vi "THzTimeScan_830_PSD_TA_170222.vi"(0 "input":T1={"Step Number"=0, "Step"=0.0, "Start Position"=0.0, "Time-out"=0, "Lockin Address"="", "Short term \nAverage#"=0, 0, "ESP300 Axis"=0, "Value"="", "Delay"=0.0, "Delay2"=0.0, "savepath"=path "", "Power meter"={"ConexPSD Reference"=refnum, "error out"={"status"=FALSE, "code"=0, "source"=""}, "Component ID"=1}}) -> (1 "loop stop":bool, 2 "x-axis":sgl[](array[numeric]), 3 "y-axis":dbl[](array[numeric]), 4 "ext. out":cluster{dbl[], dbl[], dbl[], dbl[], string[]})   [LabVIEW 2010]
uses:
  <vilib>/Utility/file.llb/Write To Spreadsheet File (string).vi
  C:/Users/THzTDS/Desktop/Align_monitoring2/THz Time(ILS7265_ESPx2_CONEXAGP_nPt_Shot202_2Pt_PSD)_LGS/Dll/Newport.CONEXPSD.CommandInterface.DLL
panel:
  out "Y pos.":dbl
  out "X pos.":dbl
  out "Pow.":dbl
  out "Y position":dbl(graph)
  out "X position":dbl(graph)
  out "Power":dbl(graph)
  out "Array":dbl[](array[numeric])
  out "String":string
  out "Read position":bool
  out "Ask position":bool
  out "Move delay":bool
  out "Read830":bool
  out "Command":string
  out "THz Signal Graph":dbl(graph)
  in  "loop stop":bool
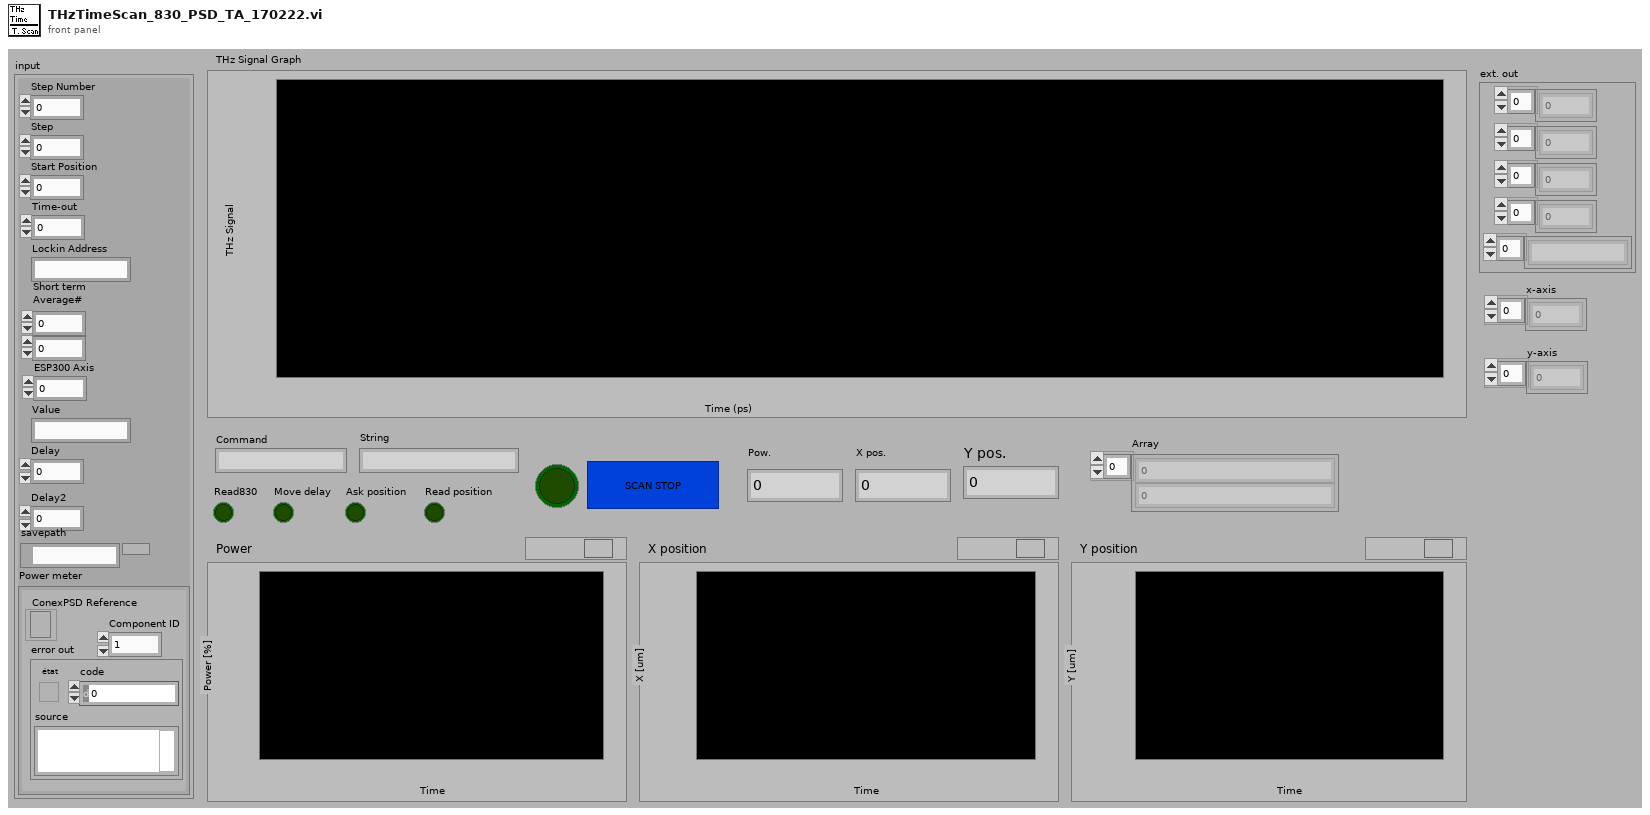
[diagram p1: front panel]
types:
  T1 = cluster{"Step Number":i32, "Step":sgl, "Start Position":sgl, "Time-out":i32, "Lockin Address":string, "Short term \nAverage#":i8, i32, "ESP300 Axis":i8, "Value":string, "Delay":dbl, "Delay2":dbl, "savepath":path, "Power meter":cluster{"ConexPSD Reference":refnum<k24>, "error out":errorcluster, "Component ID":i32}}
  T2 = cluster{"ConexPSD Reference":refnum<k24>, "error out":errorcluster, "Component ID":i32}
  T3 = cluster{"PositionX":dbl, "PositionY":dbl, "LaserPower":dbl}
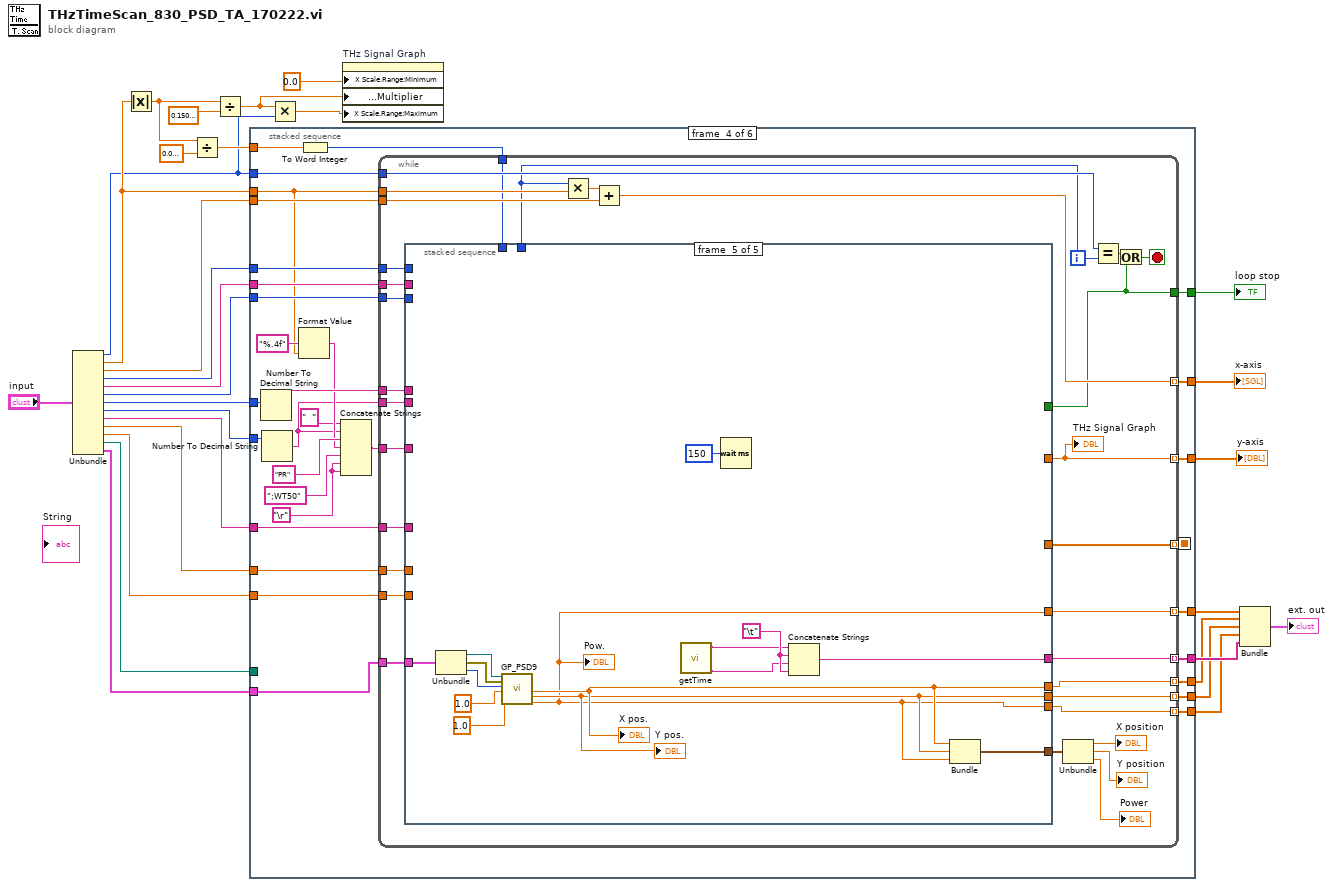
[diagram p0: block diagram]
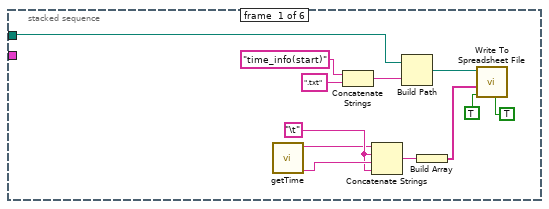
[diagram p2: hidden frame]
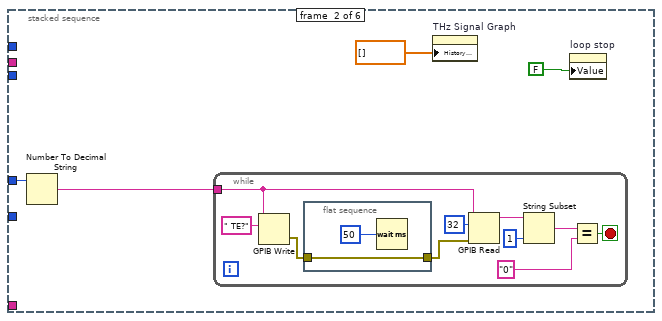
[diagram p3: hidden frame]
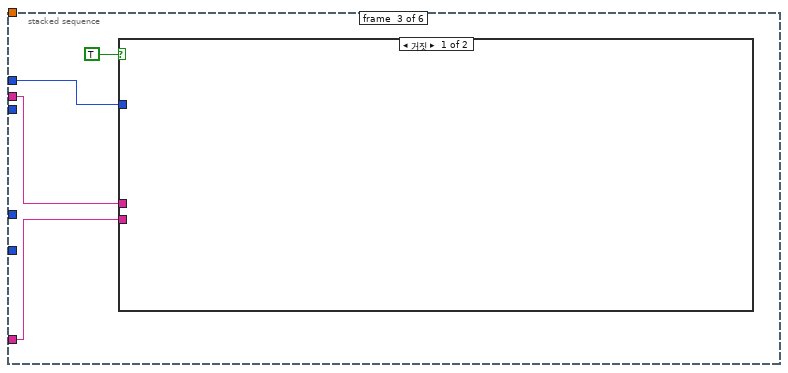
[diagram p4: hidden frame]
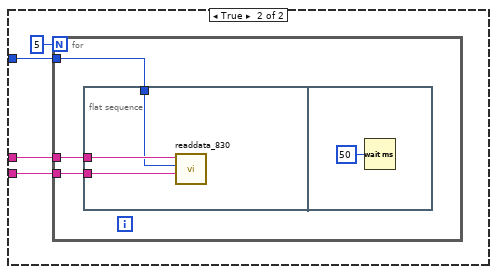
[diagram p5: hidden frame]
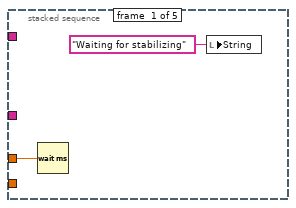
[diagram p6: hidden frame]
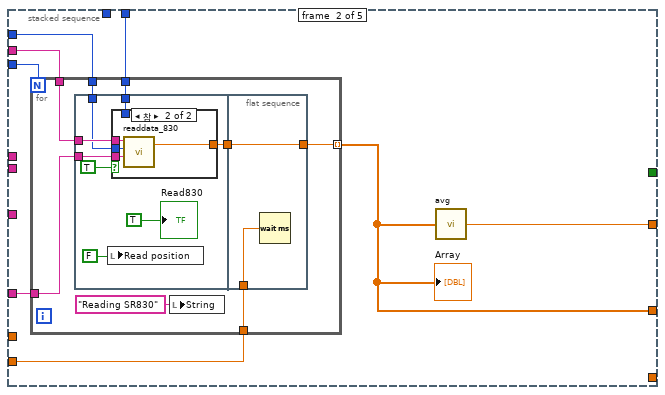
[diagram p7: hidden frame]
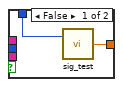
[diagram p8: hidden frame]
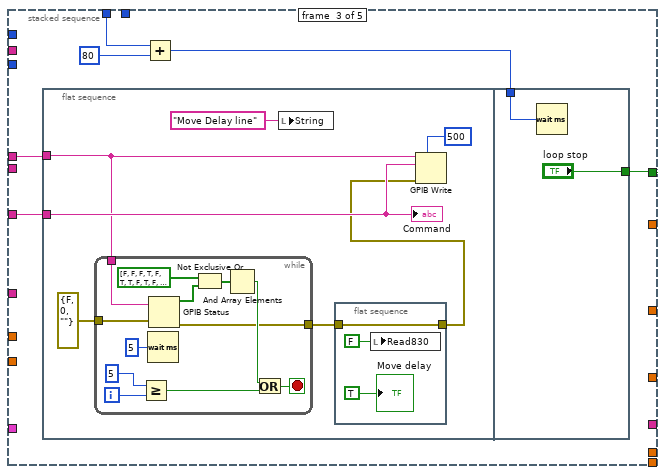
[diagram p9: hidden frame]
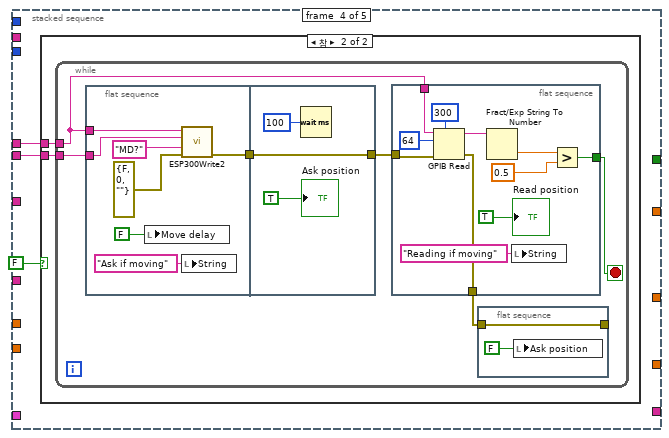
[diagram p10: hidden frame]
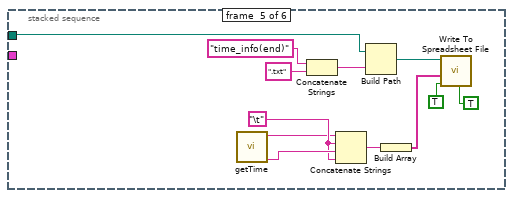
[diagram p12: hidden frame]
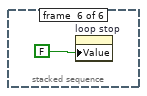
[diagram p13: hidden frame]
diagram:
  n1 = Unbundle("input") -> ("Step Number"=w2:i32, "Step"=w23:sgl, "Start Position"=w22:sgl, "Time-out"=w21:i32, "Lockin Address"=w20:string, "Short term \nAverage#"=w13:i8, w19:i32, "ESP300 Axis"=w18:i8, "Value"=w17:string, "Delay"=w12:dbl, "Delay2"=w11:dbl, "savepath"=w10:path, "Power meter"=w9:T2)
  n2 = Absolute Value(x=w23) -> (abs(x)=w26:sgl)
  n3 = Divide(x=w26, y=sgl 0.004) -> (x/y=w24:sgl)
  n4 = Divide(x=w26, y=sgl 0.15) -> (x/y=w15:sgl)
  n5 = stacked-sequence {
    seq-local: [_ _ _ w81 _ _] -> [_ _ _ _ _ _]
    tunnel: w22 -> [_ _ _ w105 _ _]
    tunnel: w21 -> [_ _ w62 w104 _ _]
    tunnel: w20 -> [_ _ w61 w103 _ _]
    tunnel: w13 -> [_ _ _ w102 _ _]
    tunnel: w19 -> [_ w44 _ w97 _ _]
    tunnel: w18 -> [_ _ _ w95 _ _]
    tunnel: w17 -> [_ _ w60 w87 _ _]
    tunnel: [_ _ _ w101 _ _] -> w30
    tunnel: [_ _ _ w100 _ _] -> w29
    tunnel: [_ _ _ w99 _ _] -> w28
    tunnel: w23 -> [_ _ _ w93 _ _]
    tunnel: w2 -> [_ _ _ w98 _ _]
    tunnel: w24 -> [_ _ _ w92 _ _]
    tunnel: w12 -> [_ _ _ w83 _ _]
    tunnel: w11 -> [_ _ _ w82 _ _]
    tunnel: w10 -> [w31 _ _ _ w250 _]
    tunnel: w9 -> [_ _ _ w79 _ _]
    tunnel: [_ _ _ w78 _ _] -> w8
    tunnel: [_ _ _ w77 _ _] -> w7
    tunnel: [_ _ _ w76 _ _] -> w6
    tunnel: [_ _ _ w75 _ _] -> w5
    tunnel: [_ _ _ w74 _ _] -> w4
    frame #0 {
      w34 = "\t"
      n6 = call "getTime.vi"() -> ("시간"=w35:string, "날짜"=w33:string)  [unwired: 10 in]
      n7 = Concatenate Strings("time_info(start)" ("string"), ".txt" ("string")) -> (w41:string)
      n8 = Concatenate Strings(w33, w34, w35, w34) -> (w32:string)
      n9 = Build Path(base path=w31, name or relative path=w41) -> (appended path=w38:path)
      n10 = Build Array(w32) -> (w37:string[])
      n11 = call-poly <vilib>:"Write To Spreadsheet File.vi"("transpose? (no:F)"=TRUE ("transpose?\n(no:F)"), "append to file? (new file:F)"=TRUE ("transpose?\n(no:F)"), "1D data"=w37, "file path (dialog if empty)"=w38) -> ()  [unwired: 4 in, 1 out]
    }
    frame #1 {
      n12 = Number To Decimal String(number=w44) -> (decimal integer string=w43:string)  [unwired: 1 in]
      n13 = while {
        tunnel: w43 -> [w49]
        stop <- w54 stop-if-true
        n14 = GPIB Write(0:w49, 1:" TE?" ("data")) -> (6:w48:errorcluster)  [unwired: 3 in, 1 out]
        n15 = flat-sequence {
          tunnel: w48 -> [w58]
          tunnel: [w58] -> w47
          frame #0 {
            n16 = Wait (ms)(milliseconds to wait=u32 50) -> ()  [unwired: 1 out]
          }
        }
        n17 = GPIB Read(0:w49, 1:32 ("byte count"), 3:w47) -> (5:w53:string)  [unwired: 2 in, 2 out]
        n18 = String Subset(string=w53, length (rest)=1 ("offset (0)")) -> (substring=w51:string)  [unwired: 1 in]
        n19 = Equal?(x=w51, y="0") -> (x = y?=w54:bool)
      }
      n20 = property on="THz Signal Graph" class="WFChart (엄격한)"("History Data"=dbl[] []) -> ()  [unwired: 2 in, 2 out]
      n21 = property on="loop stop" class="Bool (엄격한)"("Value"=FALSE) -> ()  [unwired: 2 in, 2 out]
    }
    frame #2 {
      n22 = case shown="거짓" TRUE {
        tunnel: w62 -> [_ w65]
        tunnel: w61 -> [_ w64]
        tunnel: w60 -> [_ w63]
        frame False {
        }
        frame True {
          n23 = for {
            N: 5 -> [_]
            tunnel: w64 -> [w69]
            tunnel: w63 -> [w68]
            tunnel: w65 -> [w67]
            n24 = flat-sequence {
              tunnel: w69 -> [w72]
              tunnel: w68 -> [w71]
              tunnel: w67 -> [w70]
              frame #0 {
                n25 = call "readdata_830.vi"("Command"=w71, "timeout"=w70, "Lockin Address"=w72) -> ()  [unwired: 1 in, 2 out]
              }
              frame #1 {
                n26 = Wait (ms)(milliseconds to wait=u32 50) -> ()  [unwired: 1 out]
              }
            }
          }
        }
      }
    }
    frame #3 {
      w86 = "\r"
      n27 = Number To Decimal String(number=w97) -> (decimal integer string=w96:string)  [unwired: 1 in]
      n28 = Number To Decimal String(number=w95) -> (decimal integer string=w84:string)  [unwired: 1 in]
      n29 = Format Value(format string="%.4f", value (0)=w93) -> (output string=w89:string)  [unwired: 1 in]
      n30 = To Word Integer(number=w92) -> (16bit integer=w91:i16)
      n31 = Concatenate Strings("  " ("string"), w84, "PR" ("Substring"), w89, ";WT50" ("string"), w86, w86) -> (w80:string)
      n32 = while {
        tunnel: [w121] -> w101
        tunnel: [w127] -> w99 mode=indexing
        tunnel: [w133] -> w100 mode=indexing
        tunnel: w98 -> [w132]
        tunnel: w93 -> [w131]
        tunnel: w105 -> [w130]
        tunnel: w104 -> [w122]
        tunnel: w103 -> [w129]
        tunnel: w102 -> [w128]
        tunnel: w96 -> [w126]
        tunnel: w80 -> [w125]
        tunnel: w91 -> [w124]
        tunnel: w87 -> [w123]
        tunnel: w84 -> [w120]
        tunnel: w83 -> [w119]
        tunnel: w82 -> [w118]
        tunnel: [w117] -> w81 mode=indexing
        tunnel: w79 -> [w115]
        tunnel: [w114] -> w75 mode=indexing
        tunnel: [w113] -> w76 mode=indexing
        tunnel: [w112] -> w74 mode=indexing
        tunnel: [w111] -> w78 mode=indexing
        tunnel: [w110] -> w77 mode=indexing
        i -> [w116]
        stop <- w136 stop-if-true
        n33 = stacked-sequence {
          tunnel: w129 -> [_ w143 _ _ _]
          tunnel: [_ w145 _ _ _] -> w127
          tunnel: w128 -> [_ w146 _ _ _]
          tunnel: w126 -> [_ _ w175 w203 _]
          tunnel: w125 -> [_ _ w176 _ _]
          tunnel: w124 -> [_ _ w174 _ _]
          tunnel: w123 -> [_ w144 _ _ _]
          tunnel: w122 -> [_ w142 _ _ _]
          tunnel: [_ _ w171 _ _] -> w121
          tunnel: w120 -> [_ _ _ w202 _]
          tunnel: w119 -> [w138 _ _ _ _]
          tunnel: w118 -> [_ w141 _ _ _]
          tunnel: [_ w140 _ _ _] -> w117
          tunnel: w116 -> [_ w139 _ _ _]
          tunnel: w115 -> [_ _ _ _ w241]
          tunnel: [_ _ _ _ w237] -> w111
          tunnel: [_ _ _ _ w240] -> w110
          tunnel: [_ _ _ _ w239] -> w113
          tunnel: [_ _ _ _ w238] -> w114
          tunnel: [_ _ _ _ w237] -> w112
          tunnel: [_ _ _ _ w236] -> w109
          frame #0 {
            n34 = Wait (ms)(milliseconds to wait=w138) -> ()  [unwired: 1 out]
            n35 = local write "String"("Waiting for stabilizing" ("String")) -> ()
          }
          frame #1 {
            n36 = for {
              N: w146 -> [_]
              tunnel: w143 -> [w151]
              tunnel: w142 -> [w154]
              tunnel: [w153] -> w140 mode=indexing
              tunnel: w144 -> [w152]
              tunnel: w141 -> [w148]
              tunnel: w139 -> [w147]
              n37 = flat-sequence {
                tunnel: w154 -> [w158]
                tunnel: w152 -> [w159]
                tunnel: w151 -> [w160]
                tunnel: [w157] -> w149
                tunnel: w147 -> [w155]
                tunnel: [w170] -> w153
                tunnel: w149 -> [w170]
                tunnel: w148 -> [w169]
                frame #0 {
                  n38 = local write "Read position"(FALSE ("Read position")) -> ()
                  n39 = case shown="참" TRUE {
                    tunnel: w160 -> [_ w168]
                    tunnel: w159 -> [_ w167]
                    tunnel: w158 -> [_ w166]
                    tunnel: [w164 w165] -> w157
                    tunnel: w155 -> [w163 _]
                    frame False {
                      n40 = call "sig_test.vi"("index (row)"=w163) -> ("element"=w164:dbl)  [unwired: 1 in]
                    }
                    frame True {
                      n41 = call "readdata_830.vi"("Command"=w167, "timeout"=w166, "Lockin Address"=w168) -> ("Data"=w165:dbl)  [unwired: 1 in, 1 out]
                    }
                  }
                  "Read830" <- TRUE ("Read830")
                }
                frame #1 {
                  n42 = Wait (ms)(milliseconds to wait=w169) -> ()  [unwired: 1 out]
                }
              }
              n43 = local write "String"("Reading SR830" ("String")) -> ()
            }
            "Array" <- w140
            n44 = call "avg.vi"("Array"=w140) -> ("Numeric"=w145:dbl)
          }
          frame #2 {
            n45 = flat-sequence {
              tunnel: w176 -> [w183]
              tunnel: w175 -> [w181]
              tunnel: w173 -> [w199]
              tunnel: ["loop stop"] -> w171
              frame #0 {
                n46 = while {
                  tunnel: errorcluster {"status"=FALSE, "code"=0, "source"=""} ("error in (no error)") -> [w198]
                  tunnel: [w188] -> w178
                  tunnel: w181 -> [w187]
                  i -> [w197]
                  stop <- w194 stop-if-true
                  n47 = Greater Or Equal?(x=5, y=w197) -> (x >= y?=w195:bool)
                  n48 = Wait (ms)(milliseconds to wait=u32 5) -> ()  [unwired: 1 out]
                  n49 = GPIB Status(0:w187, 1:w198) -> (2:w192:bool[], 5:w188:errorcluster)  [unwired: 2 out]
                  n50 = Not Exclusive Or(1:w192, 2:bool[] [FALSE, FALSE, FALSE, TRUE, FALSE, TRUE, TRUE, FALSE, TRUE, FALSE, FALSE, FALSE, FALSE, FALSE, FALSE, FALSE] ("status 2")) -> (0:w191:bool[])
                  n51 = And Array Elements(Boolean array=w191) -> (logical AND=w190:bool)
                  n52 = Or(x=w190, y=w195) -> (x .or. y?=w194:bool)
                }
                n53 = local write "String"("Move Delay line" ("String")) -> ()
                n54 = flat-sequence {
                  tunnel: [w186] -> w179
                  tunnel: w178 -> [w186]
                  frame #0 {
                    n55 = local write "Read830"(FALSE ("Read830")) -> ()
                    "Move delay" <- TRUE ("Move delay")
                  }
                }
                n56 = GPIB Write(0:w181, 1:w183, 3:w179, 4:500 ("timeout ms (488.2 global)")) -> ()  [unwired: 1 in, 2 out]
                "Command" <- w183
              }
              frame #1 {
                n57 = Wait (ms)(milliseconds to wait=w199) -> ()  [unwired: 1 out]
              }
            }
            n58 = Add(x=w174, y=i16 80) -> (x+y=w173:i16)
          }
          frame #3 {
            n59 = case shown="참" FALSE {
              tunnel: w203 -> [_ w205]
              tunnel: w202 -> [_ w204]
              frame False {
              }
              frame True {
                n60 = while {
                  tunnel: w205 -> [w207]
                  tunnel: w204 -> [w211]
                  stop <- w209 stop-if-true
                  n61 = flat-sequence {
                    tunnel: w211 -> [w225]
                    tunnel: w207 -> [w228]
                    tunnel: [w229] -> w208
                    tunnel: [w234] -> w210
                    tunnel: w208 -> [w234]
                    frame #0 {
                      n62 = local write "Move delay"(FALSE ("Move delay")) -> ()
                      n63 = call "ESP300Write2.vi"("error in (no error)"=errorcluster {"status"=FALSE, "code"=0, "source"=""}, "Command"="MD?", "ESP300 Channel"=w225, "ESP300 Address"=w228) -> ("error out"=w229:errorcluster)  [unwired: 3 in]
                      n64 = local write "String"("Ask if moving" ("String")) -> ()
                    }
                    frame #1 {
                      n65 = Wait (ms)(milliseconds to wait=u32 100) -> ()  [unwired: 1 out]
                      "Ask position" <- TRUE ("Ask position")
                    }
                  }
                  n66 = flat-sequence {
                    tunnel: w210 -> [w224]
                    tunnel: [w221] -> w209
                    tunnel: w207 -> [w217]
                    tunnel: [w215] -> w206
                    frame #0 {
                      n67 = GPIB Read(0:w217, 1:64 ("byte count"), 3:w224, 4:300 ("timeout ms (488.2 global)")) -> (5:w220:string, 7:w215:errorcluster)  [unwired: 1 in, 1 out]
                      n68 = Fract/Exp String To Number(string=w220) -> (number=w219:dbl)  [unwired: 3 in, 1 out]
                      n69 = local write "String"("Reading if moving" ("String")) -> ()
                      n70 = Greater?(x=w219, y=0.5) -> (0:w221:bool)
                      "Read position" <- TRUE ("Read position")
                    }
                  }
                  n71 = flat-sequence {
                    tunnel: [w213] -> _
                    tunnel: w206 -> [w213]
                    frame #0 {
                      n72 = local write "Ask position"(FALSE ("Ask position")) -> ()
                    }
                  }
                }
              }
            }
          }
          frame #4 {
            w244 = "\t"
            n73 = Unbundle(w241) -> ("ConexPSD Reference"=w249:refnum<k24>, "error out"=w248:errorcluster, "Component ID"=w247:i32)
            n74 = call "GP_PSD9.vi"("ConexPSD Reference"=w249, "error out"=w248, "Component ID"=w247, "Adress"=1.0, "shot average"=1.0) -> ("PositionX"=w239:dbl, "PositionY"=w238:dbl, "LaserPower"=w237:dbl)  [unwired: 8 in, 4 out]
            "Pow." <- w237
            "X pos." <- w239
            "Y pos." <- w238
            n75 = call "getTime.vi"() -> ("시간"=w242:string, "날짜"=w243:string)  [unwired: 10 in]
            n76 = Wait (ms)(milliseconds to wait=u32 150) -> ()  [unwired: 1 out]
            n77 = Concatenate Strings(w243, w244, w242, w244) -> (w240:string)
            n78 = Bundle("PositionX"=w239, "PositionY"=w238, "LaserPower"=w237) -> (w236:T3)  [unwired: 1 in]
          }
        }
        "THz Signal Graph" <- w127
        n79 = Multiply(x=w116, y=w131) -> (x*y=w134:sgl)
        n80 = Add(x=w134, y=w130) -> (x+y=w133:sgl)
        n81 = Unbundle(w109) -> ("PositionX"=→"X position":dbl, "PositionY"=→"Y position":dbl, "LaserPower"=→"Power":dbl)
        n82 = Equal?(x=w132, y=w116) -> (x = y?=w135:bool)
        n83 = Or(x=w135, y=w121) -> (x .or. y?=w136:bool)
      }
    }
    frame #4 {
      w253 = "\t"
      n84 = call "getTime.vi"() -> ("시간"=w254:string, "날짜"=w252:string)  [unwired: 10 in]
      n85 = Concatenate Strings("time_info(end)" ("string"), ".txt" ("string")) -> (w260:string)
      n86 = Concatenate Strings(w252, w253, w254, w253) -> (w251:string)
      n87 = Build Path(base path=w250, name or relative path=w260) -> (appended path=w257:path)
      n88 = Build Array(w251) -> (w256:string[])
      n89 = call-poly <vilib>:"Write To Spreadsheet File.vi"("transpose? (no:F)"=TRUE ("transpose?\n(no:F)"), "append to file? (new file:F)"=TRUE ("transpose?\n(no:F)"), "1D data"=w256, "file path (dialog if empty)"=w257) -> ()  [unwired: 4 in, 1 out]
    }
    frame #5 {
      n90 = property on="loop stop" class="Bool (엄격한)"("Value"=FALSE) -> ()  [unwired: 2 in, 2 out]
    }
  }
  "loop stop" <- w30
  "x-axis" <- w29
  "y-axis" <- w28
  n91 = Multiply(x=w15, y=w2) -> (x*y=w14:sgl)
  n92 = property on="THz Signal Graph" class="WFChart (엄격한)"("X Scale.Range:Minimum"=0.0, "X Scale.Offset and Multiplier:Multiplier"=w15, "X Scale.Range:Maximum"=w14) -> ()  [unwired: 2 in, 2 out]
  n93 = Bundle(w8, w6, w5, w4, w7) -> (→"ext. out":cluster{dbl[], dbl[], dbl[], dbl[], string[]})  [unwired: 1 in]
